vi "edittest decode multi-part content.vi"(8 "error in (no error)":errorcluster, 10 "Valid Content-Type: (\"text/xml\")":string="text/xml", 11 "Multi-Part Content (\"\")":string) -> (0 "error out":errorcluster, 3 "Content":string)   [LabVIEW 2011]
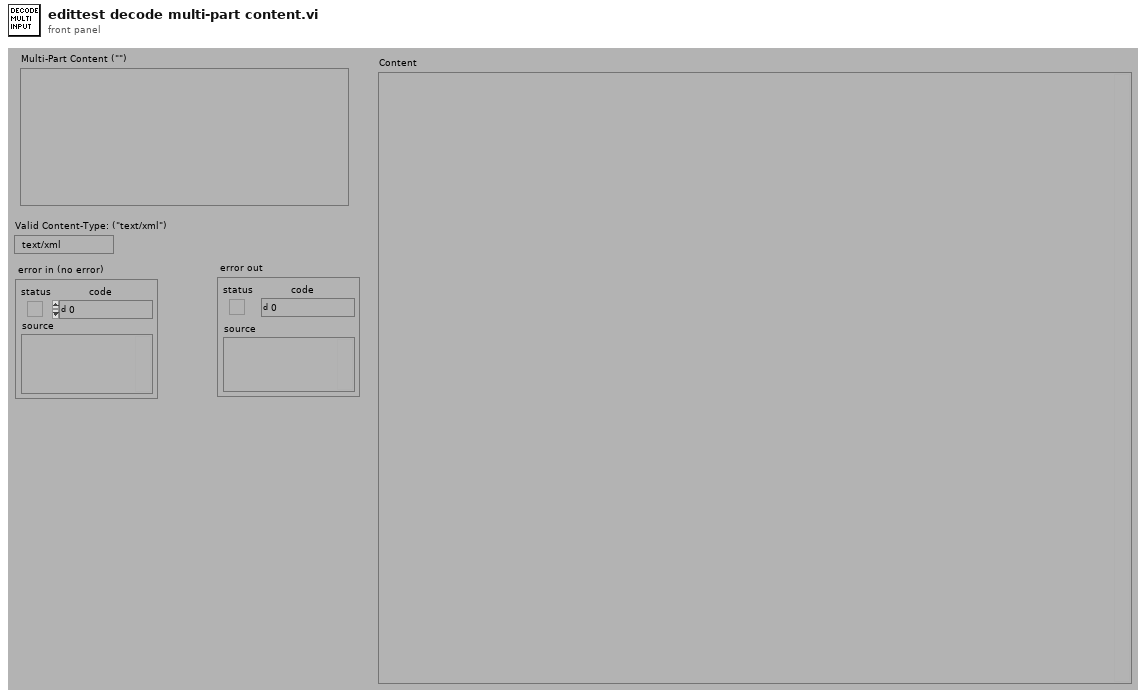
[diagram p1: front panel]
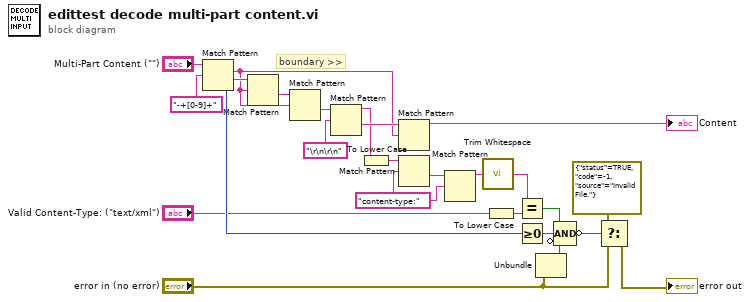
[diagram p0: block diagram]
diagram:
  w2 = "content-type:" ("regular expression")
  # "boundary >>"
  n1 = Match Pattern(string="Multi-Part Content (\"\")", regular expression="-+[0-9]+") -> (match substring=w6:string, after substring=w8:string, offset past match=w20:i32)  [unwired: 2 out]
  n2 = Match Pattern(string=w8, regular expression=w6) -> (after substring=w7:string)  [unwired: 4 out]
  n3 = Match Pattern(string=w7, regular expression=w6) -> (after substring=w5:string)  [unwired: 4 out]
  n4 = Match Pattern(string=w5, regular expression="\r\n\r\n") -> (before substring=w4:string, after substring=w22:string)  [unwired: 3 out]
  n5 = To Lower Case(string=w4) -> (all lower case string=w10:string)
  n6 = Match Pattern(string=w22, regular expression=w6) -> (before substring=→"Content":string)  [unwired: 4 out]
  n7 = Match Pattern(string=w10, regular expression=w2) -> (after substring=w3:string)  [unwired: 4 out]
  n8 = Match Pattern(string=w3, regular expression=w2) -> (before substring=w1:string)  [unwired: 4 out]
  n9 = call <vilib>:"Trim Whitespace.vi"("string"=w1) -> ("trimmed string"=w9:string)  [unwired: 1 in]
  n10 = To Lower Case(string="Valid Content-Type: (\"text/xml\")") -> (all lower case string=w14:string)
  n11 = Equal?(x=w9, y=w14) -> (x = y?=w11:bool)
  n12 = Greater Or Equal To 0?(x=w20) -> (x >= 0?=w12:bool)
  n13 = Unbundle("error in (no error)") -> ("status"=w18:bool)  [unwired: 2 out]
  n14 = Compound Arithmetic op=AND(w11, w12, invert w18) -> (invert w19:bool)
  n15 = Select(t=errorcluster {"status"=TRUE, "code"=-1, "source"="Invalid File."}, s=w19, f="error in (no error)") -> (s? t:f=→"error out":errorcluster)
